vi "snakeStep.vi"(8 "error in (no error)":errorcluster, 9 "Movement":T1, 11 "Snake in":refnum<class "Snake.lvclass">) -> (0 "error out":errorcluster, 3 "Snake out":refnum<class "Snake.lvclass">)   [LabVIEW 2014, in "Snake.lvclass"]
uses:
  Snake.lvclass
  TypeDefs/SnakeMovements.ctl
  Snake.lvclass/Snake.ctl
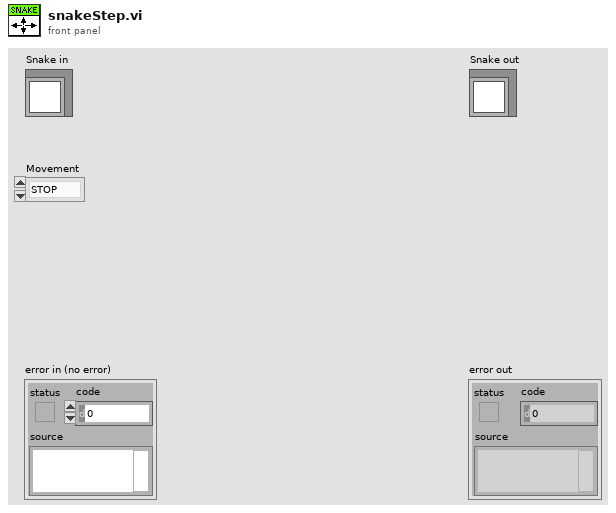
[diagram p1: front panel]
types:
  T1 = typedef "SnakeMovements.ctl" = enum16{"STOP", "UP", "DOWN", "RIGHT", "LEFT"}
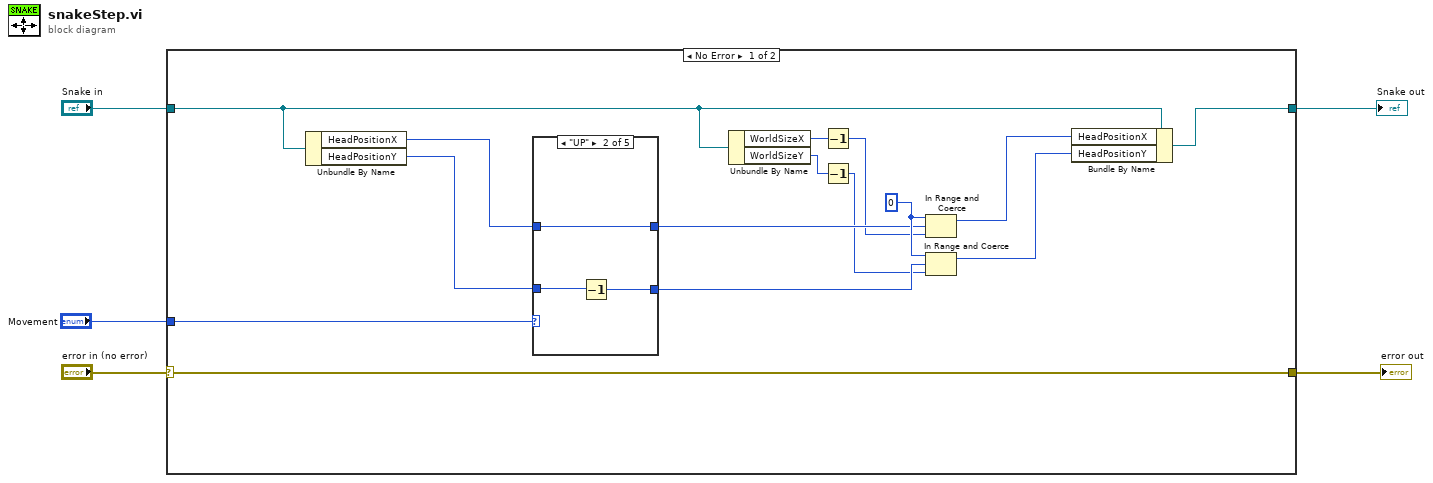
[diagram p0: block diagram]
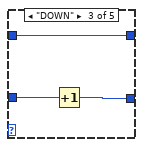
[diagram p3: hidden frame]
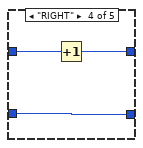
[diagram p4: hidden frame]
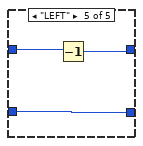
[diagram p5: hidden frame]
diagram:
  n1 = case shown="No Error" "error in (no error)" {
    selector: "error in (no error)" -> [w20 w36]
    tunnel: [w20 w36] -> w4
    tunnel: [w10 w35] -> w2
    tunnel: "Snake in" -> [w13 w35]
    tunnel: "Movement" -> [w18 _]
    frame No Error {
      w19 = 0 ("upper limit")
      n2 = Unbundle By Name(w13) -> ("HeadPositionX"=w12:i32, "HeadPositionY"=w11:i32)
      n3 = case shown="\"UP\"" w18 {
        tunnel: w12 -> [w22 w23 w26 w31 w34]
        tunnel: w11 -> [w21 w25 w28 w30 w32]
        tunnel: [w21 w24 w27 w30 w32] -> w16
        tunnel: [w22 w23 w26 w29 w33] -> w17
        frame "STOP", Default {
        }
        frame "UP" {
          n4 = Decrement(x=w25) -> (x-1=w24:i32)
        }
        frame "DOWN" {
          n5 = Increment(x=w28) -> (x+1=w27:i32)
        }
        frame "RIGHT" {
          n6 = Increment(x=w31) -> (x+1=w29:i32)
        }
        frame "LEFT" {
          n7 = Decrement(x=w34) -> (x-1=w33:i32)
        }
      }
      n8 = Unbundle By Name(w13) -> ("WorldSizeX"=w15:i32, "WorldSizeY"=w14:i32)
      n9 = Decrement(x=w15) -> (x-1=w7:i32)
      n10 = Decrement(x=w14) -> (x-1=w6:i32)
      n11 = In Range and Coerce(upper limit=w19, x=w17, lower limit=w7) -> (coerced(x)=w9:i32)  [unwired: 1 out]
      n12 = In Range and Coerce(upper limit=w19, x=w16, lower limit=w6) -> (coerced(x)=w8:i32)  [unwired: 1 out]
      n13 = Bundle By Name(cluster=w13, "HeadPositionX"=w9, "HeadPositionY"=w8) -> (w10:refnum<class "Snake.lvclass">)
    }
    frame Error {
    }
  }
  "error out" <- w4
  "Snake out" <- w2
